vi "Read Current Logic Outputs DVR.vi"(8 "error in (no error)":errorcluster, 11 "LogicIO in":refnum<class "LogicIO.lvclass">) -> (0 "error out":errorcluster, 2 "Current Logic Outputs DVR":refnum<data-value>, 3 "LogicIO out":refnum<class "LogicIO.lvclass">)   [LabVIEW 2016, in "Hardware.lvlib" / "LogicIO.lvlib" / "LogicIO.lvclass"]
uses:
  <userlib>/Common Components/Hardware/LogicIO/LogicIO/LogicIO.lvclass
  <userlib>/Common Components/Hardware/LogicIO/LogicIO/LogicIO.lvclass/LogicIO.ctl
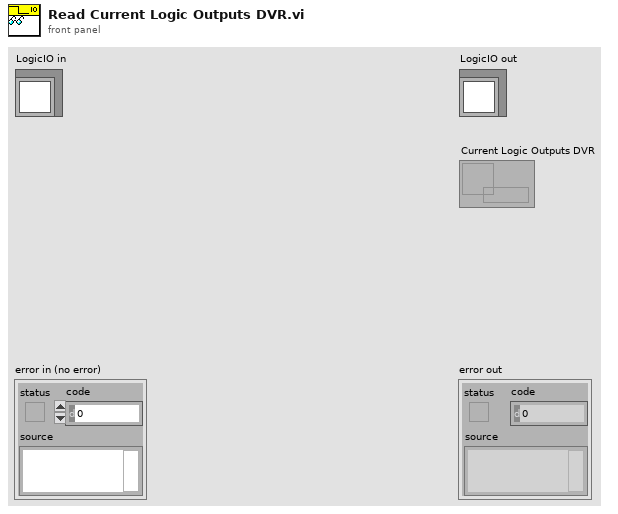
[diagram p1: front panel]
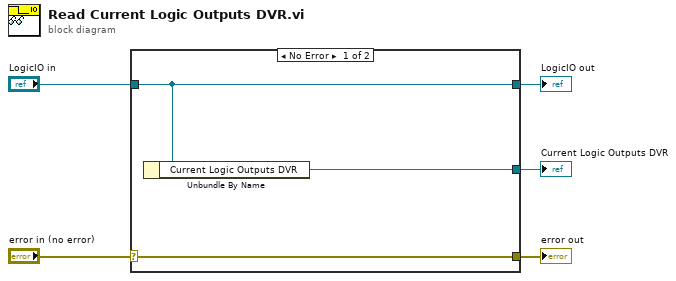
[diagram p0: block diagram]
diagram:
  n1 = case shown="No Error" "error in (no error)" {
    selector: "error in (no error)" -> [w8 w9]
    tunnel: [w8 w9] -> w4
    tunnel: [w7 w10] -> w2
    tunnel: "LogicIO in" -> [w7 w10]
    tunnel: [w6 _] -> w1
    frame No Error {
      n2 = Unbundle By Name(w7) -> ("Current Logic Outputs DVR"=w6:refnum<data-value>)
    }
    frame Error {
    }
  }
  "error out" <- w4
  "LogicIO out" <- w2
  "Current Logic Outputs DVR" <- w1
